vi "Hitrap_DiagnosticBoxGUI.set color.vi"(0 "button":refnum<vi>, 3 "Numeric":i32, 5 "error in (no error)":errorcluster) -> (19 "error out":errorcluster)   [LabVIEW 2014, in "Hitrap_DiagnosticBoxGUI.lvlib"]
doc: "copy from set color of boolean (UtilityLib)."
uses:
  Hitrap_DiagnosticBoxGUI.lvlib
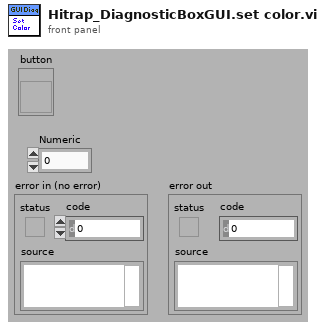
[diagram p1: front panel]
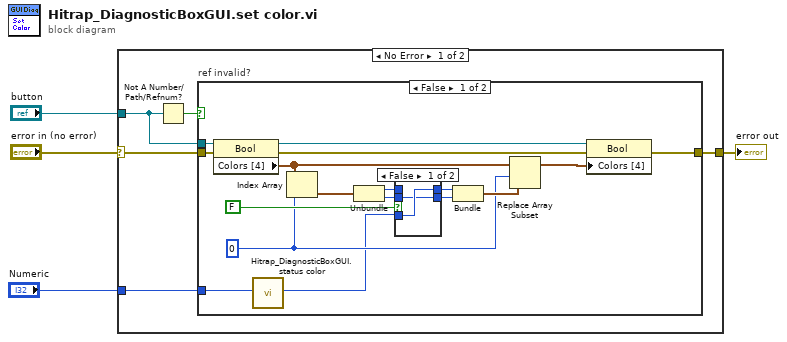
[diagram p0: block diagram]
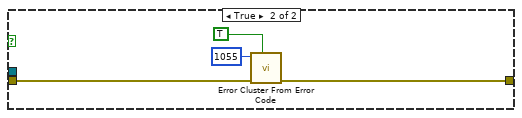
[diagram p3: hidden frame]
diagram:
  n1 = case shown="No Error" "error in (no error)" {
    selector: "error in (no error)" -> [w5 w35]
    tunnel: [w9 w35] -> w4
    tunnel: "Numeric" -> [w7 _]
    tunnel: "button" -> [w6 _]
    frame No Error {
      n2 = Not A Number/Path/Refnum?(number/path/refnum=w6) -> (NaN/Path/Refnum?=w8:bool)
      n3 = case "ref invalid?" shown="False" w8 {
        tunnel: [w26 w33] -> w9
        tunnel: w5 -> [w24 w34]
        tunnel: w6 -> [w25 _]
        tunnel: w7 -> [w11 _]
        frame False {
          w12 = 0 ("nOfPair (0)")
          n4 = property class="Bool"(reference=w25, error in=w24) -> (reference out=w23:refnum<vi>, error out=w22:errorcluster, "Colors [4]"=w20:cluster{u32, u32}[])
          n5 = call "Hitrap_DiagnosticBoxGUI.status color.vi"("Status"=w11) -> ("Color"=w10:u32)  [unwired: 18 in]
          n6 = Index Array(array=w20, index=w12) -> (element=w21:cluster{u32, u32})
          n7 = Unbundle(w21) -> (w16:u32, w14:u32)
          n8 = case shown="False" FALSE ("setTRUEColor (FALSE)") {
            tunnel: w10 -> [w28 w30]
            tunnel: [w27 w30] -> w17
            tunnel: [w28 w29] -> w15
            tunnel: w16 -> [_ w29]
            tunnel: w14 -> [w27 _]
            frame False {
            }
            frame True {
            }
          }
          n9 = Bundle("Color"=w15, "Color"=w17) -> (w19:cluster{"Color":u32, "Color":u32})  [unwired: 1 in]
          n10 = Replace Array Subset(array=w20, new element=w19, index=w12) -> (w18:cluster{u32, u32}[])
          n11 = property class="Bool"(reference=w23, error in=w22, "Colors [4]"=w18) -> (error out=w26:errorcluster)  [unwired: 1 out]
        }
        frame True {
          n12 = call <vilib>:"Error Cluster From Error Code.vi"("show call chain? (False)"=TRUE, "error in (no error)"=w34, "error code (0)"=1055) -> ("error out"=w33:errorcluster)  [unwired: 6 in]
        }
      }
    }
    frame Error {
    }
  }
  "error out" <- w4
